vi "Review Queues.vi"() -> ()   [LabVIEW 2024, in "Application.lvlib"]
uses:
  Application.lvlib
  Support/General Type Defs/Queue Message.ctl
  Modules/Session Scanner/Scanner Queue - Get.vi
  Modules/User Interface/UI Queue - Get.vi
  Modules/Session Scanner/Session Scanner.lvlib
  Modules/User Interface/User Interface.lvlib
  Support/General Type Defs/General Type Defs.lvlib
panel:
  out "UI elements":T1[](array[typedef])
  out "UI elements":T1[](array[typedef])
  in  "Stop":bool
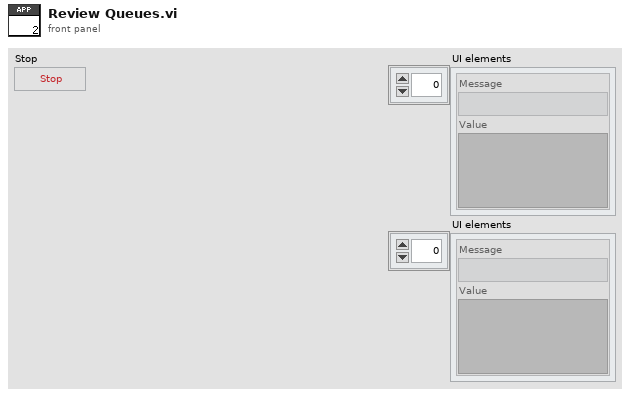
[diagram p1: front panel]
types:
  T1 = typedef "General Type Defs.lvlib/Queue Message.ctl" = cluster{"Message":string, "Value":variant}
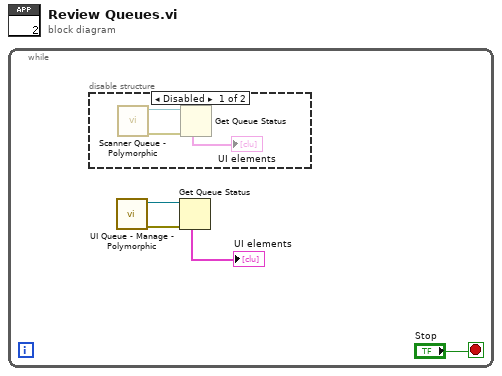
[diagram p0: block diagram]
diagram:
  n1 = while {
    stop <- "Stop" stop-if-true
    n2 = disable-structure shown="Disabled" {
      frame Disabled {
        n3 = call-poly "Scanner Queue - Polymorphic.vi"() -> ("error out"=w6:errorcluster, "queue out"=w7:refnum<queue>)  [unwired: 10 in]
        n4 = Get Queue Status(queue=w7, error in (no error)=w6) -> (elements=→"UI elements":T1[])  [unwired: 1 in, 7 out]
      }
      frame Enabled {
      }
    }
    n5 = call-poly "UI Queue - Manage - Polymorphic.vi"() -> ("error out"=w2:errorcluster, "queue out"=w3:refnum<queue>)  [unwired: 10 in]
    n6 = Get Queue Status(queue=w3, error in (no error)=w2) -> (elements=→"UI elements":T1[])  [unwired: 1 in, 7 out]
  }
